vi "Unflatten Alpha.vi"(1 "image data":T1) -> (0 "32-bit pixmap":u32[][](array[numeric]))   [LabVIEW 2023, in "Glyph Drawer.lvlib" / "Glyph Source.lvclass"]
uses:
  Glyph Source.lvclass
  <vilib>/picture/picture.llb/imagedata.ctl
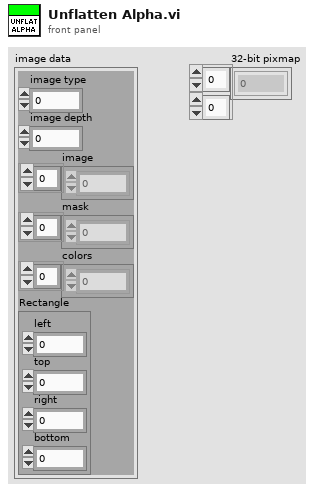
[diagram p1: front panel]
types:
  T1 = typedef "imagedata.ctl" = cluster{"image type":i32, "image depth":i32, "image":u8[], "mask":u8[], "colors":u32[], "Rectangle":cluster{"left":i16, "top":i16, "right":i16, "bottom":i16}}
  T2 = cluster{"left":i16, "top":i16, "right":i16, "bottom":i16}
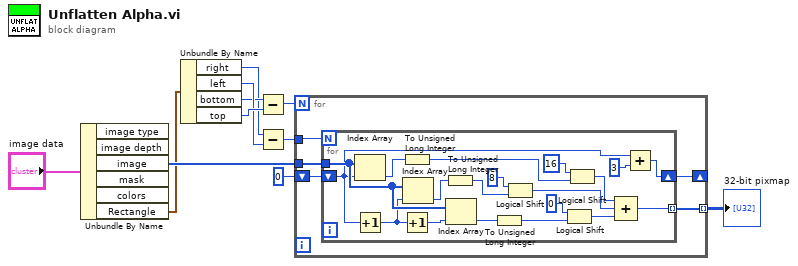
[diagram p0: block diagram]
diagram:
  n1 = Unbundle By Name("image data") -> ("image"=w9:u8[], "Rectangle"=w8:T2)  [unwired: 4 out]
  n2 = Unbundle By Name(w8) -> ("right"=w2:i16, "left"=w6:i16, "bottom"=w3:i16, "top"=w7:i16)
  n3 = Subtract(x=w3, y=w7) -> (x-y=w5:i16)
  n4 = Subtract(x=w2, y=w6) -> (x-y=w4:i16)
  n5 = for {
    N: w5 -> [_]
    tunnel: w4 -> [w12]
    tunnel: w9 -> [w16]
    tunnel: [w15] -> w11 mode=indexing
    shift-right: [w13] -> _
    shift-left: 0 -> [w14]
    n6 = for {
      N: w12 -> [_]
      tunnel: w16 -> [w35]
      tunnel: [w25] -> w15 mode=indexing
      shift-right: [w23] -> w13
      shift-left: w14 -> [w22]
      n7 = Index Array(array=w35, index=w22) -> (element=w28:u8)
      n8 = Increment(x=w22) -> (x+1=w21:i32)
      n9 = To Unsigned Long Integer(number=w28) -> (unsigned 32bit integer=w18:u32)
      n10 = Increment(x=w21) -> (x+1=w34:i32)
      n11 = Index Array(array=w35, index=w21) -> (element=w20:u8)
      n12 = To Unsigned Long Integer(number=w20) -> (unsigned 32bit integer=w31:u32)
      n13 = Index Array(array=w35, index=w34) -> (element=w29:u8)
      n14 = To Unsigned Long Integer(number=w29) -> (unsigned 32bit integer=w30:u32)
      n15 = Logical Shift(y=i8 8, x=w31) -> (x << y=w27:u32)
      n16 = Logical Shift(y=i8 0, x=w30) -> (x << y=w26:u32)
      n17 = Logical Shift(y=i8 16, x=w18) -> (x << y=w17:u32)
      n18 = Compound Arithmetic op=ADD(w17, w27, w26) -> (w25:u32)
      n19 = Add(x=w22, y=3) -> (x+y=w23:i32)
    }
  }
  "32-bit pixmap" <- w11
